vi "LOG_AsyncHandler.vi"(8 "error in (no error)":errorcluster, 11 "Message queue in":refnum<queue>) -> (0 "error out":errorcluster)   [LabVIEW 2015]
uses:
  Controls/LOG_MessageQueue.ctl
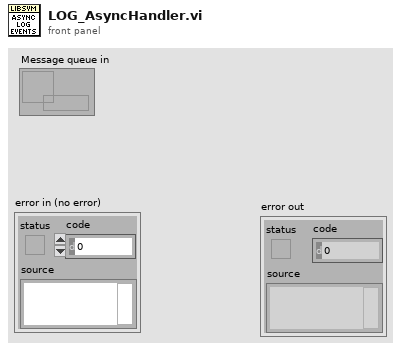
[diagram p1: front panel]
types:
  T1 = typedef "LOG_MessageQueue.ctl" = cluster{"Time":timestamp, "message":string}
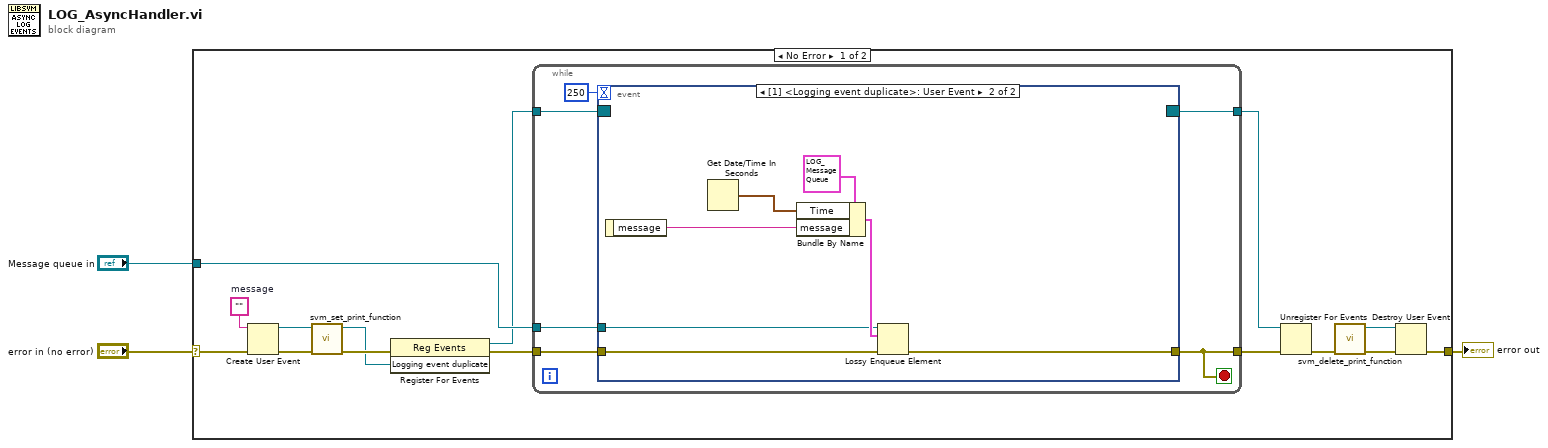
[diagram p0: block diagram]
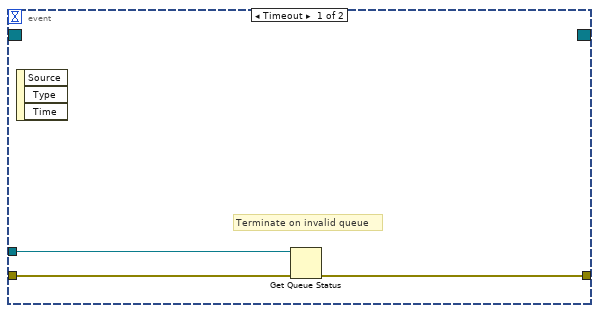
[diagram p2: hidden frame]
diagram:
  n1 = case shown="No Error" "error in (no error)" {
    selector: "error in (no error)" -> [w10 w35]
    tunnel: [w14 w35] -> w3
    tunnel: "Message queue in" -> [w15 _]
    frame No Error {
      w6 = ""  # message
      n2 = Create User Event(user event datatype=w6, error in=w10) -> (user event=w5:refnum<user-event>, error out=w8:errorcluster)
      n3 = call "svm_set_print_function.vi"("error in (no error)"=w8, "Logging event"=w5) -> ("error out"=w9:errorcluster, "Logging event duplicate"=w4:refnum<user-event>)  [unwired: 8 in]
      n4 = register-events(error in=w9, w4) -> (reference out=w7:refnum<event-registration>, error out=w18:errorcluster)  [unwired: 1 in]
      n5 = while {
        tunnel: w18 -> [w24]
        tunnel: [w23] -> w17
        tunnel: [w21] -> w16
        tunnel: w15 -> [w20]
        tunnel: w7 -> [w19]
        stop <- w23 stop-if-true
        n6 = event shown="[1] <Logging event duplicate>: User Event" {
          selector: w19 -> [_ _]
          dyn-events: [_ _] -> w21
          timeout: 250 -> [_ _]
          tunnel: w24 -> [w27 w34]
          tunnel: [w26 w33] -> w23
          tunnel: w20 -> [w25 w29]
          event Timeout {
            # "Terminate on invalid queue"
            n7 = event-data() -> ()  [unwired: 1 in, 3 out]
            n8 = Get Queue Status(queue=w25, error in (no error)=w27) -> (error out=w26:errorcluster)  [unwired: 1 in, 7 out]
          }
          event User Event {
            n9 = event-data() -> ("message"=w28:string)  [unwired: 1 in]
            n10 = Get Date/Time In Seconds() -> (seconds since 1Jan1904=w30:timestamp)
            n11 = Bundle By Name(cluster=T1 {"Time"=timestamp(0 s since 1904-01-01), "message"=""} ("Log Event"), "Time"=w30, "message"=w28) -> (w31:T1)
            n12 = Lossy Enqueue Element(queue=w29, element=w31, error in (no error)=w34) -> (error out=w33:errorcluster)  [unwired: 3 out]
          }
        }
      }
      n13 = Unregister For Events(event registration refnum=w16, error in=w17) -> (error out=w13:errorcluster)
      n14 = call "svm_delete_print_function.vi"("error in (no error)"=w13) -> ("error out"=w12:errorcluster, "User Event Out"=w11:refnum<user-event>)  [unwired: 9 in]
      n15 = Destroy User Event(user event=w11, error in=w12) -> (error out=w14:errorcluster)
    }
    frame Error {
    }
  }
  "error out" <- w3
